vi "CAN Message to Floats.vi"(10 "CAN Message":u8[](array[numeric])) -> (1 "Float_1":sgl, 2 "Float_0":sgl)   [LabVIEW 2019]
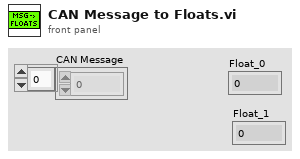
[diagram p1: front panel]
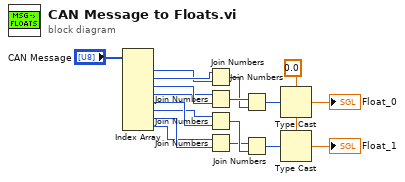
[diagram p0: block diagram]
diagram:
  w3 = sgl 0.0 ("y")
  n1 = Index Array(array="CAN Message") -> (element #1=w17:u8, element #2=w18:u8, element #3=w16:u8, element #4=w15:u8, element #5=w8:u8, element #6=w7:u8, element #7=w6:u8, element #8=w5:u8)  [unwired: 8 in]
  n2 = Join Numbers(hi=w18, lo=w17) -> ((hi.lo)=w13:u16)
  n3 = Join Numbers(hi=w15, lo=w16) -> ((hi.lo)=w14:u16)
  n4 = Join Numbers(hi=w7, lo=w8) -> ((hi.lo)=w10:u16)
  n5 = Join Numbers(hi=w5, lo=w6) -> ((hi.lo)=w9:u16)
  n6 = Join Numbers(hi=w14, lo=w13) -> ((hi.lo)=w12:u32)
  n7 = Join Numbers(hi=w9, lo=w10) -> ((hi.lo)=w4:u32)
  n8 = Type Cast(type=w3, x=w12) -> (*(type *) &x=→"Float_0":sgl)
  n9 = Type Cast(type=w3, x=w4) -> (*(type *) &x=→"Float_1":sgl)
